vi "saveControl.vi"(8 "error in (no error)":errorcluster, 11 "Topic in":refnum<class "Topic.lvclass">) -> (0 "error out":errorcluster, 3 "Topic out":refnum<class "Topic.lvclass">)   [LabVIEW 2012, in "Topic.lvclass"]
uses:
  Topic.lvclass
  Topic.lvclass/Topic.ctl
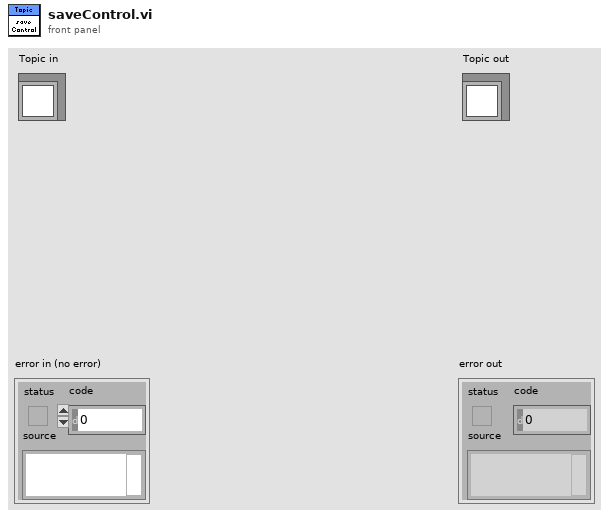
[diagram p1: front panel]
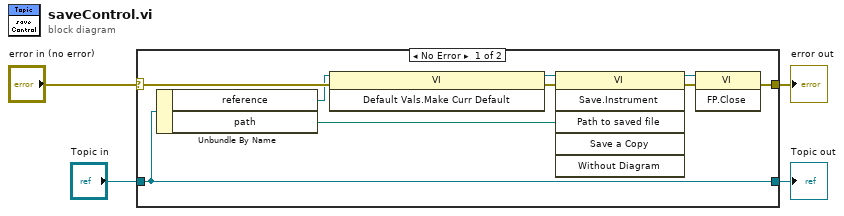
[diagram p0: block diagram]
diagram:
  n1 = case shown="No Error" "error in (no error)" {
    selector: "error in (no error)" -> [w7 w15]
    tunnel: [w10 w15] -> w3
    tunnel: [w13 w14] -> w1
    tunnel: "Topic in" -> [w13 w14]
    frame No Error {
      n2 = Unbundle By Name(w13) -> ("reference"=w6:refnum<vi>, "path"=w5:path)
      n3 = invoke class="VI" method="Default Vals.Make Curr Default"(reference=w6, error in=w7) -> (reference out=w9:refnum<vi>, error out=w8:errorcluster)  [unwired: 1 in, 1 out]
      n4 = invoke class="VI" method="Save.Instrument"(reference=w9, error in=w8, "Path to saved file"=w5) -> (reference out=w12:refnum<vi>, error out=w11:errorcluster)  [unwired: 3 in, 4 out]
      n5 = invoke class="VI" method="FP.Close"(reference=w12, error in=w11) -> (error out=w10:errorcluster)  [unwired: 1 in, 2 out]
    }
    frame Error {
    }
  }
  "error out" <- w3
  "Topic out" <- w1
